vi "Release-hardware.vi"(8 "error in (no error)":errorcluster, 11 "Data ref. in":refnum<data-value>) -> (0 "error out":errorcluster, 3 "Data ref.":refnum<data-value>)   [LabVIEW 2013, in "CameraVision.lvlib" / "CV-Main.lvclass"]
uses:
  CV-Main.lvclass
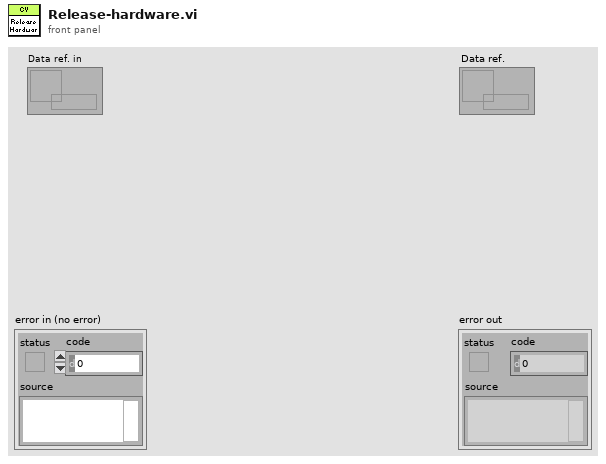
[diagram p1: front panel]
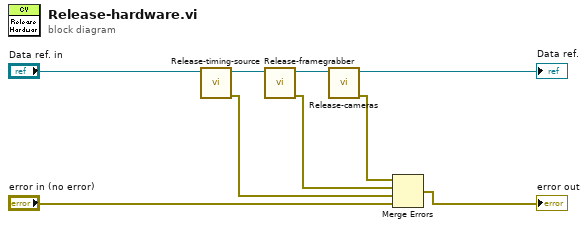
[diagram p0: block diagram]
diagram:
  n1 = call "Release-timing-source.vi"("Data ref. in"="Data ref. in") -> ("error IO"=w7:errorcluster, "Data ref."=w5:refnum<data-value>)  [unwired: 9 in]
  n2 = call "Release-framegrabber.vi"("Data ref. in"=w5) -> ("error IO"=w1:errorcluster, "Data ref."=w4:refnum<data-value>)  [unwired: 9 in]
  n3 = call "Release-cameras.vi"("Data ref. in"=w4) -> ("error IO"=w2:errorcluster, "Data ref."=→"Data ref.":refnum<data-value>)  [unwired: 9 in]
  n4 = Merge Errors(w2, w1, w7, "error in (no error)") -> (→"error out":errorcluster)
